vi "XOR.vi"(1 "b":bool, 2 "a":bool) -> (0 "x":bool)   [LabVIEW 2012]
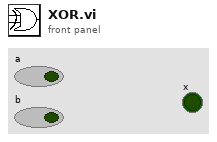
[diagram p1: front panel]
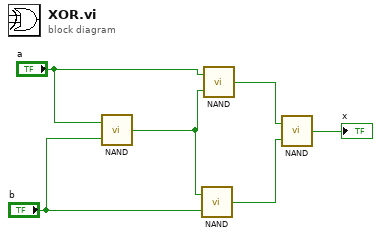
[diagram p0: block diagram]
diagram:
  n1 = call "NAND.vi"("b"="b", "a"="a") -> ("x"=w4:bool)
  n2 = call "NAND.vi"("b"="b", "a"=w4) -> ("x"=w2:bool)
  n3 = call "NAND.vi"("b"=w4, "a"="a") -> ("x"=w3:bool)
  n4 = call "NAND.vi"("b"=w2, "a"=w3) -> ("x"=→"x":bool)
